vi "log2.vi"(11 "Input":dbl) -> (2 "Numeric":i32, 3 "Boolean":bool)   [LabVIEW 2020]
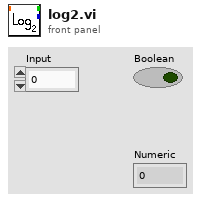
[diagram p1: front panel]
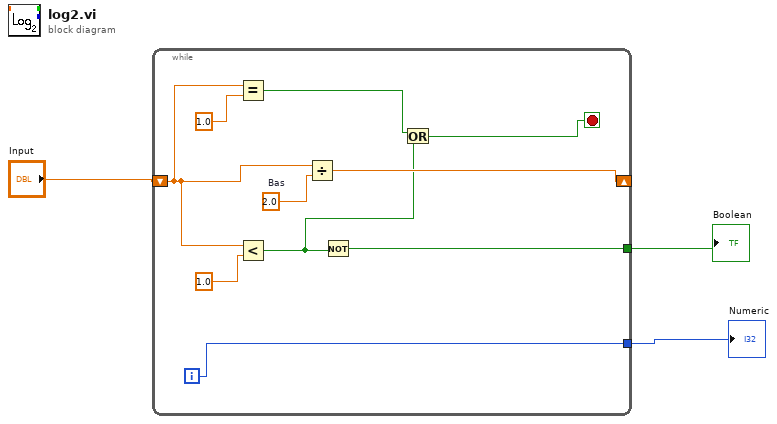
[diagram p0: block diagram]
diagram:
  n1 = while {
    shift-right: [w10] -> _
    shift-left: "Input" -> [w9]
    tunnel: [w13] -> w3
    tunnel: [w7] -> w2
    i -> [w13]
    stop <- w4 stop-if-true
    w11 = 2.0  # Bas
    n2 = Equal?(x=w9, y=1.0) -> (x = y?=w6:bool)
    n3 = Less?(x=w9, y=1.0) -> (x < y?=w5:bool)
    n4 = Divide(x=w9, y=w11) -> (x/y=w10:dbl)
    n5 = Not(x=w5) -> (.not. x?=w7:bool)
    n6 = Or(x=w6, y=w5) -> (x .or. y?=w4:bool)
  }
  "Numeric" <- w3
  "Boolean" <- w2
